vi "Resync with ni-xnet channels.vi"(8 "Error In":errorcluster, 11 "Device Item Ref in in":T1 format="%.0x") -> (0 "Error Out":errorcluster, 3 "Device Item Ref out":T1 format="%.0x")   [LabVIEW 2018, in "NI-XNET Monitor System Explorer.lvlib"]
uses:
  NI-XNET Monitor System Explorer.lvlib
  <vilib>/NI Veristand/Custom Device API/Custom Device Item Ref.ctl
  <vilib>/NI Veristand/Custom Device Tools/Custom Device Utility Library/Search Direction.ctl
  Shared/Constants.vi
  <vilib>/NI Veristand/Custom Device Tools/Custom Device Utility Library/NI VeriStand - Search for Item by GUID.vi
  <vilib>/NI Veristand/Custom Device Tools/Custom Device Utility Library/NI VeriStand - Search for Item by Property.vi
  <vilib>/NI Veristand/Custom Device Tools/Custom Device Utility Library/Custom Device Utility Library.lvlib
  Shared/NI-XNET Monitor Shared.lvlib
  <vilib>/NI Veristand/Custom Device API/Custom Device API.lvlib
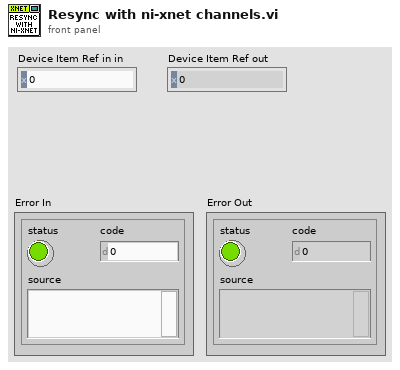
[diagram p1: front panel]
types:
  T1 = typedef "Custom Device API.lvlib/Custom Device Item Ref.ctl" = u64
  T2 = typedef "Custom Device Utility Library.lvlib/Search Direction.ctl" = enum16{"Down", "Up"}
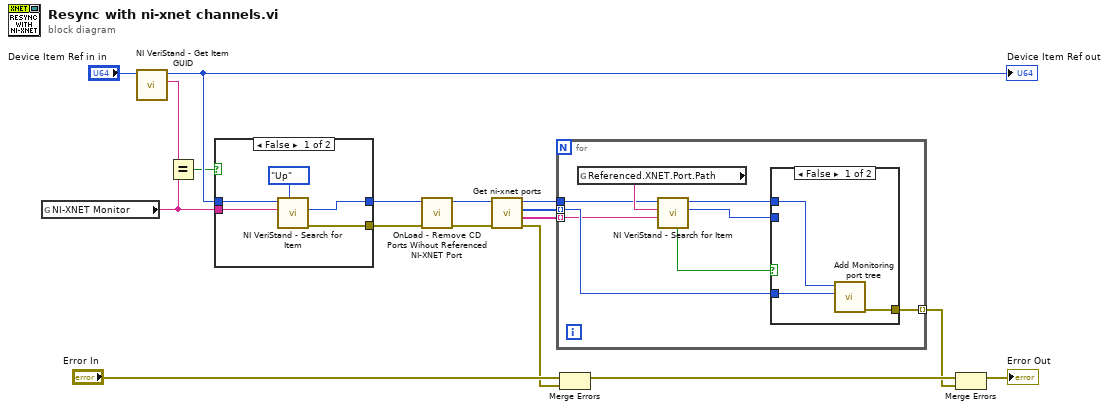
[diagram p0: block diagram]
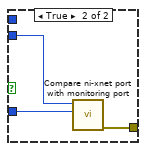
[diagram p3: hidden frame]
diagram:
  n1 = global read "Constants.vi" "NI-XNET Monitor"() -> (w12:string)
  n2 = call <vilib>:"NI VeriStand - Get Item GUID.vi"("Item Ref in"="Device Item Ref in in") -> ("GUID"=w13:string, "Item Ref out"=w14:T1)  [unwired: 8 in, 1 out]
  "Device Item Ref out" <- w14
  n3 = Equal?(x=w13, y=w12) -> (x = y?=w11:bool)
  n4 = case shown="False" w11 {
    tunnel: [w21 _] -> w6
    tunnel: [w20 w23] -> w8
    tunnel: w14 -> [w19 w23]
    tunnel: w12 -> [w18 _]
    frame False {
      n5 = call-poly <vilib>:"NI VeriStand - Search for Item.vi"("Direction (Down)"=Search_Direction."Up", "Item GUID"=w18, "Section Ref in"=w19) -> ("error out"=w21:errorcluster, "Item Ref"=w20:T1)  [unwired: 5 in, 2 out]
    }
    frame True {
    }
  }
  n6 = call "OnLoad - Remove CD Ports Wihout Referenced NI-XNET Port.vi"("error in (no error)"=w6, "Device Item Ref in in"=w8) -> ("error out"=w5:errorcluster, "Device Item Ref out"=w7:T1)  [unwired: 8 in]
  n7 = call "Get ni-xnet ports.vi"("Error In"=w5, "Device Item Ref in"=w7) -> ("Error Out"=w10:errorcluster, "NI-XNET Port Item Paths"=w3:string[], "NI-XNET Port Refs"=w4:T1[], "Device Item Ref out"=w16:T1)  [unwired: 6 in]
  n8 = for {
    tunnel: w4 -> [w27] mode=indexing
    tunnel: w16 -> [w28]
    tunnel: w3 -> [w25] mode=indexing
    tunnel: [w24] -> w1 mode=indexing
    n9 = global read "Constants.vi" "Referenced.XNET.Port.Path"() -> (w31:string)
    n10 = call-poly <vilib>:"NI VeriStand - Search for Item.vi"("Property Value"=w25, "Property Name"=w31, "Section Ref in"=w28) -> ("Item Ref"=w29:T1, "Section Ref out"=w30:T1, "Found"=w26:bool)  [unwired: 5 in, 1 out]
    n11 = case shown="False" w26 {
      tunnel: w30 -> [w34 _]
      tunnel: w29 -> [_ w37]
      tunnel: w27 -> [w33 w36]
      tunnel: [w32 w35] -> w24
      frame False {
        n12 = call "Add Monitoring port tree.vi"("NI-XNET Port (Item Ref)"=w33, "Device Item Ref in"=w34) -> ("Error Out"=w32:errorcluster)  [unwired: 8 in, 1 out]
      }
      frame True {
        n13 = call "Compare ni-xnet port with monitoring port.vi"("NI-XNET Port Item Ref In"=w36, "CD Port Item Ref In"=w37) -> ("Error Out"=w35:errorcluster)  [unwired: 7 in, 2 out]
      }
    }
  }
  n14 = Merge Errors("Error In", w10) -> (w9:errorcluster)
  n15 = Merge Errors(w9, w1) -> (→"Error Out":errorcluster)
